vi "getResult.vi"(8 "error in (no error)":errorcluster, 9 "data_shape":sgl[][](array[numeric]), 11 "InferEngineStruct":u64) -> (0 "error out":errorcluster, 1 "data out":sgl[][](array[numeric]), 3 "InferEngineStruct out":u64)   [LabVIEW 2023]
uses:
  openvino_vi_wrapper.dll
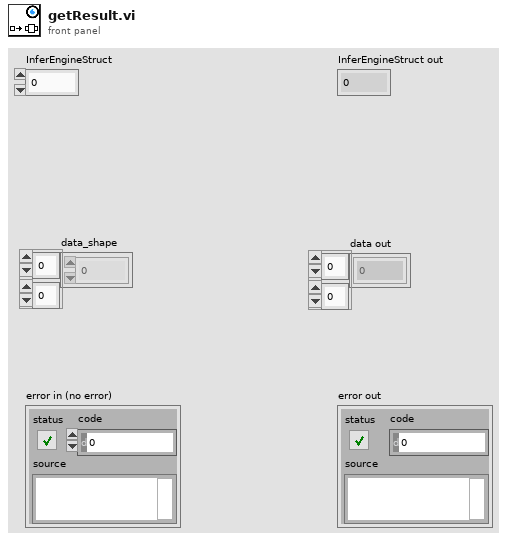
[diagram p1: front panel]
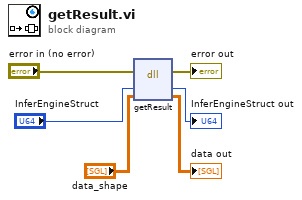
[diagram p0: block diagram]
diagram:
  n1 = dll-call lib="C:/Users/NUC/Desktop/LabVIEW_OpenVINO_Dll/yolov8_openvino_opensource/openvino_vi_wrapper/openvino_vi_wrapper.dll" fn="getResult"(error in="error in (no error)", "InferEngineStruct"="InferEngineStruct", "data"="data_shape") -> (error out=→"error out":errorcluster, "InferEngineStruct"=→"InferEngineStruct out":u64, "data"=→"data out":sgl[][])  [unwired: 3 in, 1 out]
